vi "CRYDB Insert Into AxisID.vi"(0 "connection reference":T1, 1 "Axies Name":string, 3 "error in":errorcluster) -> (7 "connection reference out":T1, 8 "Axis_ID":i32, 10 "error out":errorcluster)   [LabVIEW 2013]
uses:
  <vilib>/addons/database/Connection.llb/Conn ObjectReference.ctl
  <vilib>/addons/database/Auxilliary.llb/DB Tools Column Info.ctl
  <vilib>/addons/database/Auxilliary.llb/DB Tools DataTypes.ctl
  <vilib>/addons/database/Connection.llb/Conn Execute.vi
  <vilib>/addons/database/Recordset.llb/Rec Fetch Recordset Data (R).vi
  <vilib>/addons/database/Recordset.llb/Rec Destroy - Connection.vi
  <vilib>/addons/database/_DB Variant To Data/Database Variant To Data.xnode
  <vilib>/addons/database/NI_Database_API.lvlib
panel:
  in  "Table":cluster{"Axis_ID":u32, "Axis_Name":string}
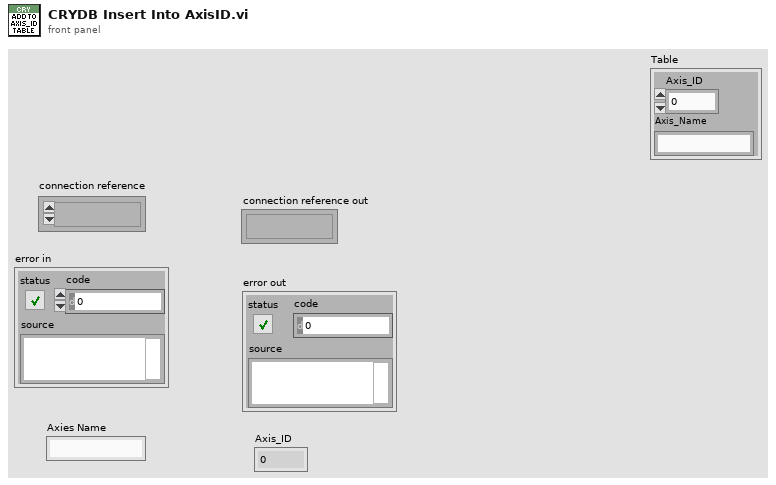
[diagram p1: front panel]
types:
  T1 = typedef "NI_Database_API.lvlib/Conn ObjectReference.ctl" = refnum<k1>
  T2 = typedef "NI_Database_API.lvlib/DB Tools Column Info.ctl" = cluster{"column name":string, "data type":T3, "size":i32, "allow null?":bool}
  T3 = typedef "NI_Database_API.lvlib/DB Tools DataTypes.ctl" = enum16{"String", "Long (I32)", "Single (SGL)", "Double (DBL)", "Date/Time", "Binary"}
  T4 = typedef "NI_Database_API.lvlib/Rec ObjectReference.ctl" = refnum<k1>
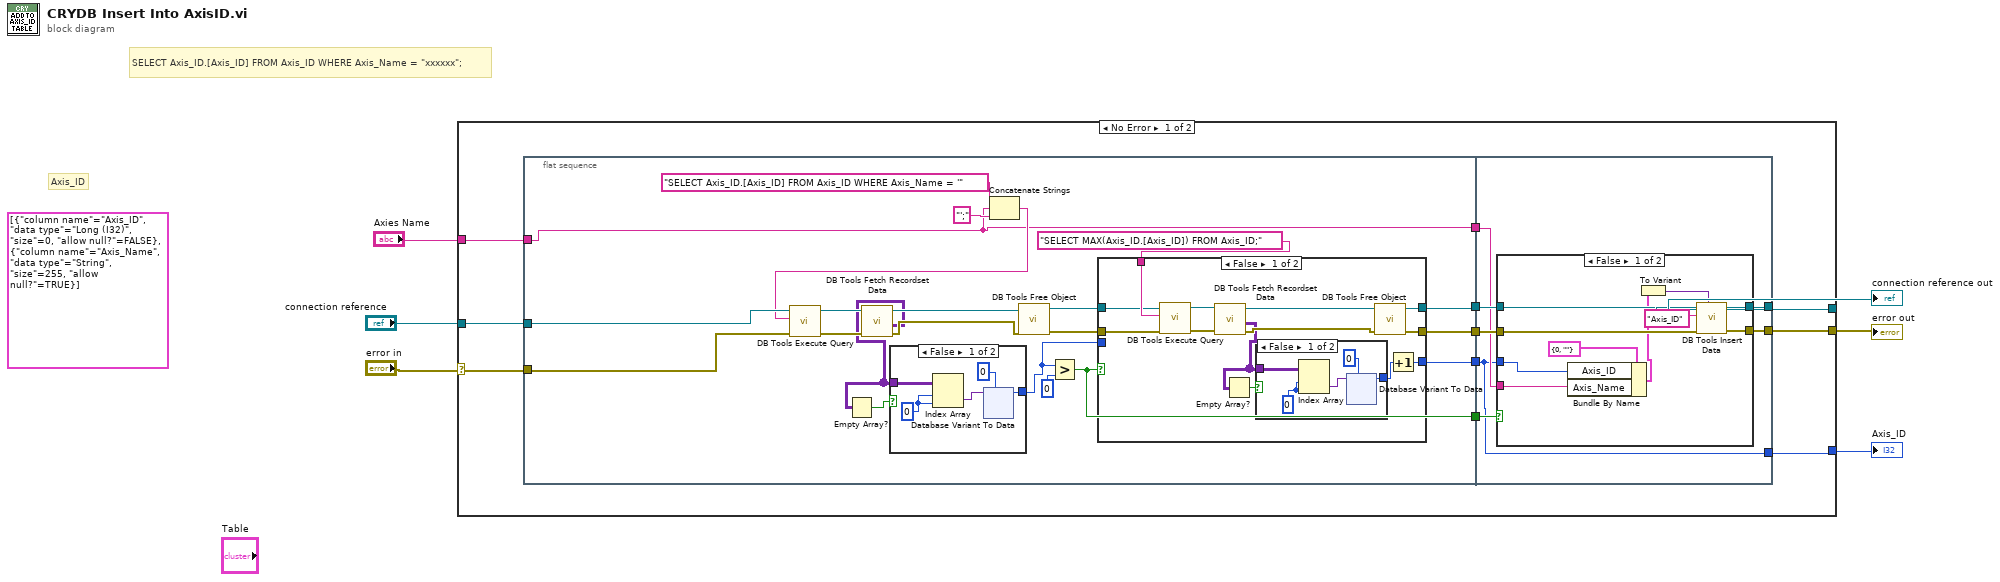
[diagram p0: block diagram]
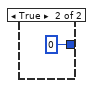
[diagram p2: hidden frame]
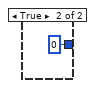
[diagram p3: hidden frame]
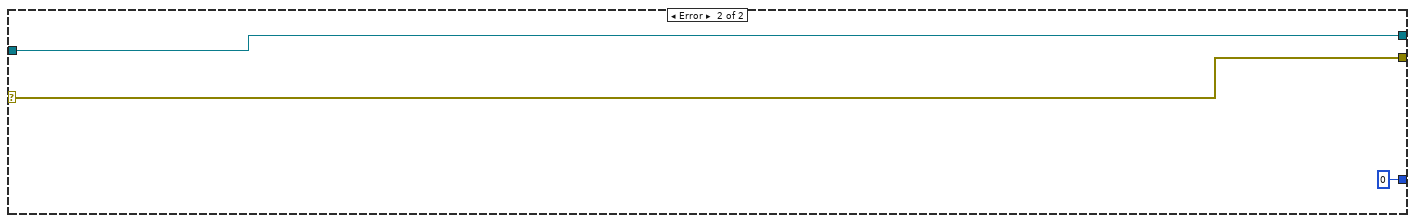
[diagram p6: hidden frame]
diagram:
  (unwired) T2[] [{"column name"="Axis_ID", "data type"=enum."Long (I32)", "size"=0, "allow null?"=FALSE}, {"column name"="Axis_Name", "data type"=enum."String", "size"=255, "allow null?"=TRUE}] ("column information")
  # "Axis_ID"
  # "SELECT Axis_ID.[Axis_ID] FROM Axis_ID WHERE Axis_Name = \"xxxxxx\";"
  n1 = case shown="No Error" "error in" {
    selector: "error in" -> [w15 w151]
    tunnel: "connection reference" -> [w17 w152]
    tunnel: [w13 w152] -> w3
    tunnel: [w12 w151] -> w4
    tunnel: [w8 0 ("data")] -> w2
    tunnel: "Axies Name" -> [w7 _]
    frame No Error {
      n2 = flat-sequence {
        tunnel: w17 -> [w38]
        tunnel: [w25] -> w16
        tunnel: w15 -> [w34]
        tunnel: [w24] -> w14
        tunnel: [w23] -> w11
        tunnel: [w22] -> w10
        tunnel: [w21] -> w9
        tunnel: w7 -> [w21]
        tunnel: w16 -> [w137]
        tunnel: w14 -> [w136]
        tunnel: [w135] -> w13
        tunnel: [w134] -> w12
        tunnel: w11 -> [w133]
        tunnel: w10 -> [w131]
        tunnel: w9 -> [w132]
        tunnel: [w131] -> w8
        frame #0 {
          n3 = Concatenate Strings("SELECT Axis_ID.[Axis_ID] FROM Axis_ID WHERE Axis_Name = '" ("SQL query"), w21, "';" ("string")) -> (w29:string)
          n4 = call-poly <vilib>:"DB Tools Execute Query.vi"("error in (no error)"=w34, "SQL query"=w29, "connection reference"=w38) -> ("error out"=w33:errorcluster, "recordset reference"=w37:T4)  [unwired: 5 in]
          n5 = call-poly <vilib>:"DB Tools Fetch Recordset Data.vi"("error in (no error)"=w33, "recordset reference"=w37) -> ("error out"=w32:errorcluster, "recordset data"=w18:variant[][], "recordset reference out"=w36:T4)  [unwired: 3 in]
          n6 = Empty Array?(array=w18) -> (empty?=w20:bool)
          n7 = case shown="False" w20 {
            tunnel: w18 -> [w43 _]
            tunnel: [w40 0 ("data")] -> w19
            frame False {
              w42 = 0 ("disabled index (col)")
              n8 = Index Array(array=w43, index (row)=w42, index (col)=w42) -> (element=w39:variant)
              n9 = xnode "Database Variant To Data"("database variant"=w39, "type"=0) -> ("data"=w40:i32)  [unwired: 1 in, 1 out]
            }
            frame True {
            }
          }
          n10 = call-poly <vilib>:"DB Tools Free Object.vi"("error in (no error)"=w32, "recordset reference"=w36) -> ("error out"=w27:errorcluster, "connection reference"=w28:T1)  [unwired: 8 in]
          n11 = Greater?(x=w19, y=0) -> (0:w23:bool)
          n12 = case shown="False" w23 {
            tunnel: w19 -> [_ w130]
            tunnel: w28 -> [w88 w129]
            tunnel: w27 -> [w87 w128]
            tunnel: "SELECT MAX(Axis_ID.[Axis_ID]) FROM Axis_ID;" ("SQL query") -> [w89 _]
            tunnel: [w84 w130] -> w22
            tunnel: [w81 w129] -> w25
            tunnel: [w80 w128] -> w24
            frame False {
              n13 = call-poly <vilib>:"DB Tools Execute Query.vi"("error in (no error)"=w87, "SQL query"=w89, "connection reference"=w88) -> ("error out"=w85:errorcluster, "recordset reference"=w86:T4)  [unwired: 5 in]
              n14 = call-poly <vilib>:"DB Tools Fetch Recordset Data.vi"("error in (no error)"=w85, "recordset reference"=w86) -> ("error out"=w82:errorcluster, "recordset data"=w77:variant[][], "recordset reference out"=w83:T4)  [unwired: 3 in]
              n15 = Empty Array?(array=w77) -> (empty?=w79:bool)
              n16 = case shown="False" w79 {
                tunnel: w77 -> [w94 _]
                tunnel: [w91 0 ("data")] -> w78
                frame False {
                  w93 = 0 ("disabled index (col)")
                  n17 = Index Array(array=w94, index (row)=w93, index (col)=w93) -> (element=w90:variant)
                  n18 = xnode "Database Variant To Data"("database variant"=w90, "type"=0) -> ("data"=w91:i32)  [unwired: 1 in, 1 out]
                }
                frame True {
                }
              }
              n19 = call-poly <vilib>:"DB Tools Free Object.vi"("error in (no error)"=w82, "recordset reference"=w83) -> ("error out"=w80:errorcluster, "connection reference"=w81:T1)  [unwired: 8 in]
              n20 = Increment(x=w78) -> (x+1=w84:i32)
            }
            frame True {
            }
          }
        }
        frame #1 {
          n21 = case shown="False" w133 {
            tunnel: w137 -> [w147 w149]
            tunnel: w136 -> [w145 w148]
            tunnel: [w143 w149] -> w135
            tunnel: [w142 w148] -> w134
            tunnel: w131 -> [w141 _]
            tunnel: w132 -> [w140 _]
            frame False {
              n22 = Bundle By Name(cluster=cluster{"Axis_ID":u32, "Axis_Name":string} {"Axis_ID"=0, "Axis_Name"=""} ("Table"), "Axis_ID"=w141, "Axis_Name"=w140) -> (w139:cluster{"Axis_ID":u32, "Axis_Name":string})
              n23 = To Variant(anything=w139) -> (Variant=w144:variant)
              n24 = call <vilib>:"DB Tools Insert Data.vi"("data"=w144, "error in (no error)"=w145, "table"="Axis_ID", "connection reference"=w147) -> ("error out"=w142:errorcluster, "connection reference out"=w143:T1)  [unwired: 6 in]
            }
            frame True {
            }
          }
        }
      }
    }
    frame Error {
    }
  }
  "connection reference out" <- w3
  "error out" <- w4
  "Axis_ID" <- w2
